vi "Modbus UI Settings.vi"() -> (0 "error out":errorcluster)   [LabVIEW 2021]
uses:
  <vilib>/Utility/config.llb/Write Key (String).vi
  <vilib>/Utility/config.llb/Write Key (U32).vi
  <vilib>/Utility/config.llb/NI_LVConfig.lvlib
panel:
  in  "Button":bool
  in  "Tab Control":enum32{"Modbus Serial", "Modbus TCP"}(tab)
  in  "Serial Port":refnum<visa-resource-name>
  in  "baud rate":u32=9600 caption="Baud Rate"
  in  "serial type":enum16{"RTU", "ASCII"}(ring) caption="Serial Type"
  in  "unit ID":u8=1 caption="Unit ID"
  in  "port":u16=502 caption="Port"
  in  "address":string caption="IP Address"
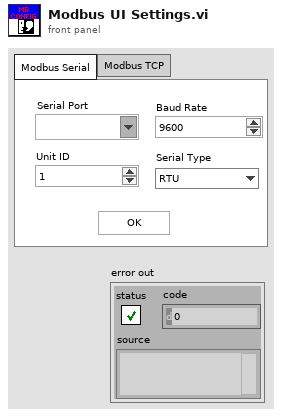
[diagram p1: front panel]
types:
  T1 = typedef "NI_LVConfig.lvlib/Config Data RefNum.ctl" = refnum<k1>
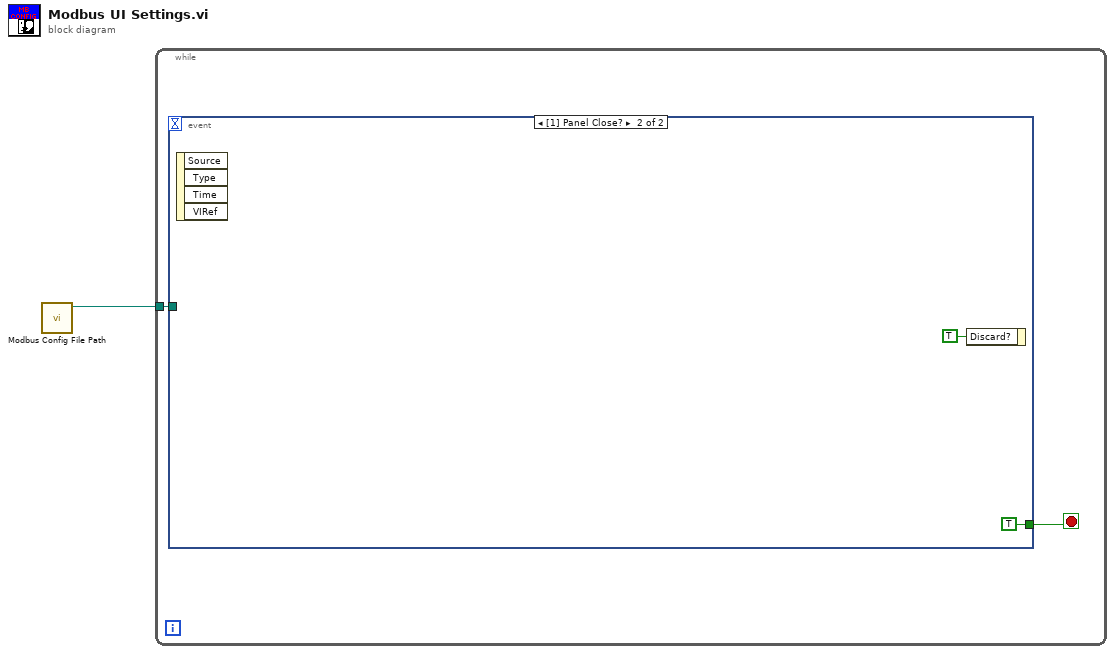
[diagram p0: block diagram]
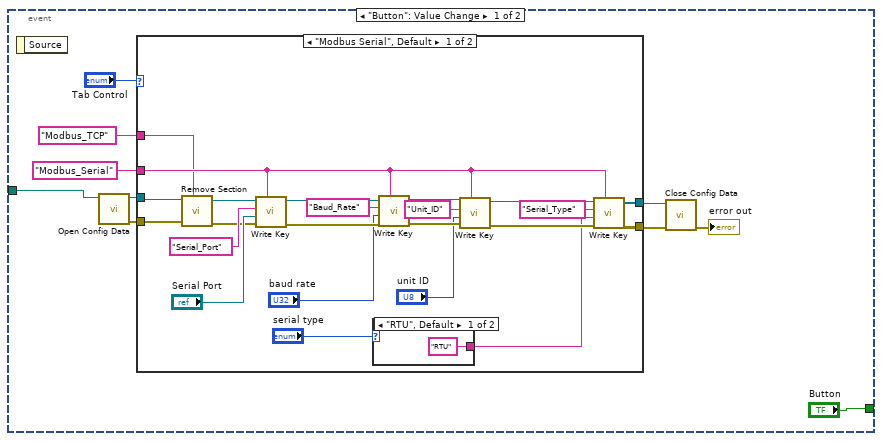
[diagram p2: hidden frame]
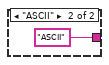
[diagram p3: hidden frame]
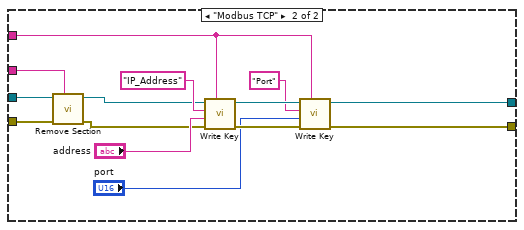
[diagram p4: hidden frame]
diagram:
  n1 = call "Modbus Config File Path.vi"() -> ("appended path out"=w1:path)  [unwired: 11 in]
  n2 = while {
    tunnel: w1 -> [w2]
    stop <- w3 stop-if-true
    n3 = event shown="[1] Panel Close?" {
      selector: _ -> [_ _]
      dyn-events: _ -> [_ _]
      timeout: _ -> [_ _]
      tunnel: ["Button" TRUE ("Button")] -> w3
      tunnel: w2 -> [w10 _]
      event "Button": Value Change {
        n4 = event-data() -> ()  [unwired: 1 in, 1 out]
        n5 = call <vilib>:"Open Config Data.vi"("configuration file path"=w10) -> ("error out"=w12:errorcluster, "refnum"=w11:T1)  [unwired: 8 in, 1 out]
        n6 = case shown="\"Modbus Serial\", Default" "Tab Control" {
          tunnel: w12 -> [w18 w44]
          tunnel: w11 -> [w15 w42]
          tunnel: [w25 w46] -> w9
          tunnel: [w22 w45] -> w8
          tunnel: "Modbus_Serial" ("section") -> [w19 w40]
          tunnel: "Modbus_TCP" ("section") -> [w14 w39]
          frame "Modbus Serial", Default {
            n7 = call <vilib>:"Remove Section.vi"("section"=w14, "error in (no error)"=w18, "refnum"=w15) -> ("error out"=w17:errorcluster, "refnum out"=w16:T1)  [unwired: 6 in, 1 out]
            n8 = call-poly <vilib>:"Write Key.vi"("section"=w19, "error in (no error)"=w17, "value"="Serial Port", "key"="Serial_Port", "refnum"=w16) -> ("error out"=w33:errorcluster, "refnum out"=w34:T1)  [unwired: 4 in, 1 out]
            n9 = case shown="\"RTU\", Default" "serial type" {
              tunnel: ["RTU" "ASCII"] -> w21
              frame "RTU", Default {
              }
              frame "ASCII" {
              }
            }
            n10 = call-poly <vilib>:"Write Key.vi"("section"=w19, "error in (no error)"=w33, "value"="baud rate", "key"="Baud_Rate", "refnum"=w34) -> ("error out"=w29:errorcluster, "refnum out"=w30:T1)  [unwired: 4 in, 1 out]
            n11 = call-poly <vilib>:"Write Key.vi"("section"=w19, "error in (no error)"=w29, "value"="unit ID", "key"="Unit_ID", "refnum"=w30) -> ("error out"=w23:errorcluster, "refnum out"=w24:T1)  [unwired: 4 in, 1 out]
            n12 = call-poly <vilib>:"Write Key.vi"("section"=w19, "error in (no error)"=w23, "value"=w21, "key"="Serial_Type", "refnum"=w24) -> ("error out"=w25:errorcluster, "refnum out"=w22:T1)  [unwired: 4 in, 1 out]
          }
          frame "Modbus TCP" {
            n13 = call <vilib>:"Remove Section.vi"("section"=w40, "error in (no error)"=w44, "refnum"=w42) -> ("error out"=w43:errorcluster, "refnum out"=w41:T1)  [unwired: 6 in, 1 out]
            n14 = call-poly <vilib>:"Write Key.vi"("section"=w39, "error in (no error)"=w43, "value"="address", "key"="IP_Address", "refnum"=w41) -> ("error out"=w51:errorcluster, "refnum out"=w52:T1)  [unwired: 4 in, 1 out]
            n15 = call-poly <vilib>:"Write Key.vi"("section"=w39, "error in (no error)"=w51, "value"="port", "key"="Port", "refnum"=w52) -> ("error out"=w46:errorcluster, "refnum out"=w45:T1)  [unwired: 4 in, 1 out]
          }
        }
        n16 = call <vilib>:"Close Config Data.vi"("error in (no error)"=w9, "refnum"=w8) -> ("error out"=→"error out":errorcluster)  [unwired: 8 in, 1 out]
      }
      event Panel Close? {
        n17 = event-data() -> ()  [unwired: 1 in, 4 out]
        n18 = event-data("Discard?"=TRUE) -> ()  [unwired: 1 in, 1 out]
      }
    }
  }
